vi "savephoto.vi"(0 "camera":u32) -> (1 "dst":u8[](array[numeric]), 2 "camera 2":u32)   [LabVIEW 2016]
uses:
  Vital supporting file for labview program/C++/Dll for liveview/x64/Debug/Dll for liveview.dll
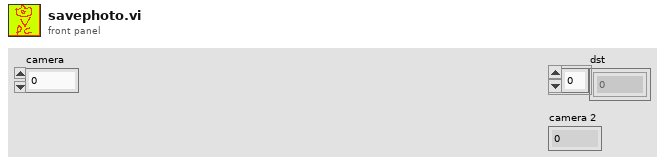
[diagram p1: front panel]
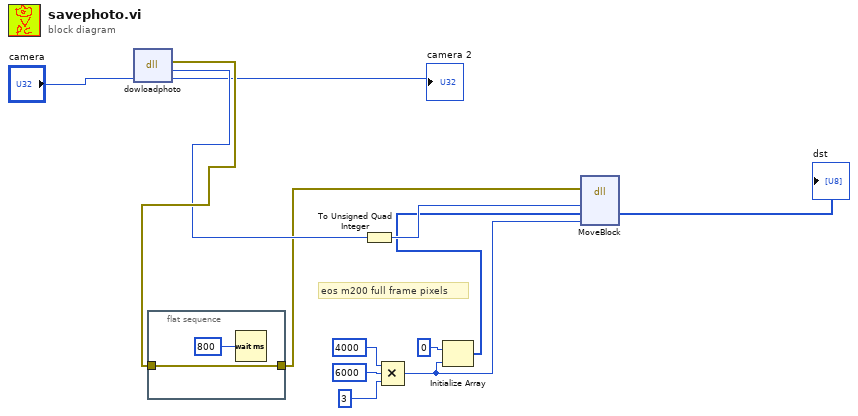
[diagram p0: block diagram]
diagram:
  # "eos m200 full frame pixels"
  n1 = dll-call lib="D:/All users/PoSheng/src/labview for canon om/Vital supporting file for labview program/C++/Dll for liveview/x64/Debug/Dll for liveview.dll" fn="dowloadphoto"("camera"="camera") -> (error out=w9:errorcluster, "return type"=w7:i64, "camera"=→"camera 2":u32)  [unwired: 3 in, 1 out]
  n2 = flat-sequence {
    tunnel: w9 -> [w15]
    tunnel: [w15] -> w6
    frame #0 {
      n3 = Wait (ms)(milliseconds to wait=u32 800) -> ()  [unwired: 1 out]
    }
  }
  n4 = To Unsigned Quad Integer(1:w7) -> (0:w8:u64)
  n5 = Compound Arithmetic op=MULTIPLY(4000 ("dimension size"), 6000 ("dimension size"), 3 ("dimension size")) -> (w5:i32)
  n6 = Initialize Array ("初始化数组")(u8 0 ("element"), w5) -> (w4:u8[])
  n7 = dll-call lib="LabVIEW" fn="MoveBlock"(error in=w6, "src"=w8, "dst"=w4, "size"=w5) -> ("dst"=→"dst":u8[])  [unwired: 5 in, 2 out]
